vi "Memory Manager Pre-Build.vi"   [LabVIEW 2016]
uses:
  Build Automation.lvlib
types:
  T1 = cluster{"Status Message":refnum<data-value>, "Progress":refnum<data-value>, "Stop":refnum<data-value>}
  T2 = enum16{"Share clones between instances", "Preallocate clone for each instance"}
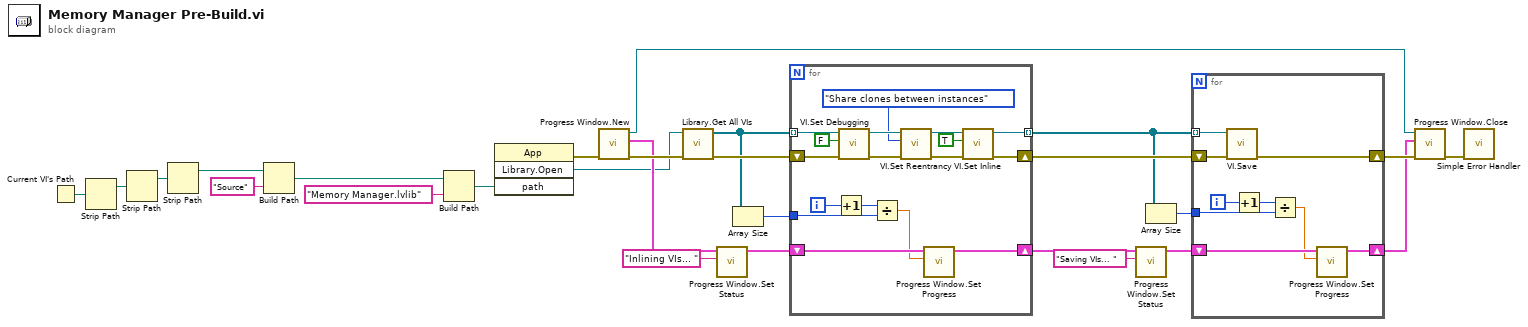
[diagram p0: block diagram]
diagram:
  n1 = Current VI's Path() -> (path=w26:path)
  n2 = Strip Path(path=w26) -> (stripped path=w25:path)  [unwired: 1 out]
  n3 = Strip Path(path=w25) -> (stripped path=w24:path)  [unwired: 1 out]
  n4 = Strip Path(path=w24) -> (stripped path=w23:path)  [unwired: 1 out]
  n5 = Build Path(base path=w23, name or relative path="Source") -> (appended path=w22:path)
  n6 = Build Path(base path=w22, name or relative path="Memory Manager.lvlib" ("library name")) -> (appended path=w20:path)
  n7 = invoke class="App" method="Library.Open"("path"=w20) -> (error out=w18:errorcluster, "Open Library"=w6:refnum<vi>)  [unwired: 3 in, 2 out]
  n8 = call "Progress Window.New.vi"("error in (no error)"=w18) -> ("error out"=w8:errorcluster, "DVRs"=w7:T1, "VI refnum"=w12:refnum<vi>)  [unwired: 8 in]
  n9 = call "Library.Get All VIs.vi"("error in (no error)"=w8, "library ref"=w6) -> ("error out"=w19:errorcluster, "vi refs"=w16:refnum<vi>[])  [unwired: 8 in]
  n10 = call "Progress Window.Set Status.vi"("Status Message"="Inlining VIs... " ("data value"), "DVRs in"=w7) -> ("DVRs out"=w14:T1)  [unwired: 8 in, 1 out]
  n11 = Array Size(array=w16) -> (size(s)=w15:i32)
  n12 = for {
    tunnel: w16 -> [w44] mode=indexing
    shift-right: [w28] -> w11
    shift-left: w19 -> [w43]
    tunnel: w15 -> [w34]
    shift-right: [w31] -> w10
    shift-left: w14 -> [w33]
    tunnel: [w29] -> w4 mode=indexing
    i -> [w36]
    n13 = Increment(x=w36) -> (x+1=w35:i32)
    n14 = call "VI.Set Debugging.vi"("error in (no error)"=w43, "Allow Debugging"=FALSE, "vi ref in"=w44) -> ("error out"=w40:errorcluster, "vi ref out"=w41:refnum<vi>)  [unwired: 7 in]
    n15 = Divide(x=w35, y=w34) -> (x/y=w32:dbl)
    n16 = call "VI.Set Reentrancy.vi"("error in (no error)"=w40, "Reentrancy Type"=T2."Share clones between instances", "vi ref in"=w41) -> ("error out"=w38:errorcluster, "vi ref out"=w39:refnum<vi>)  [unwired: 7 in]
    n17 = call "Progress Window.Set Progress.vi"("Progress"=w32, "DVRs in"=w33) -> ("DVRs out"=w31:T1)  [unwired: 8 in, 1 out]
    n18 = call "VI.Set Inline.vi"("error in (no error)"=w38, "Inline VI"=TRUE, "vi ref in"=w39) -> ("error out"=w28:errorcluster, "vi ref out"=w29:refnum<vi>)  [unwired: 7 in]
  }
  n19 = call "Progress Window.Set Status.vi"("Status Message"="Saving VIs... ", "DVRs in"=w10) -> ("DVRs out"=w5:T1)  [unwired: 8 in, 1 out]
  n20 = Array Size(array=w4) -> (size(s)=w3:i32)
  n21 = for {
    shift-right: [w51] -> w2
    shift-left: w11 -> [w53]
    tunnel: w4 -> [w52] mode=indexing
    shift-right: [w45] -> w1
    shift-left: w5 -> [w47]
    tunnel: w3 -> [w49]
    i -> [w48]
    n22 = call "VI.Save.vi"("error in (no error)"=w53, "vi ref in"=w52) -> ("error out"=w51:errorcluster)  [unwired: 8 in, 1 out]
    n23 = Increment(x=w48) -> (x+1=w50:i32)
    n24 = Divide(x=w50, y=w49) -> (x/y=w46:dbl)
    n25 = call "Progress Window.Set Progress.vi"("Progress"=w46, "DVRs in"=w47) -> ("DVRs out"=w45:T1)  [unwired: 8 in, 1 out]
  }
  n26 = call "Progress Window.Close.vi"("error in (no error)"=w2, "DVRs in"=w1, "VI refnum"=w12) -> ("error out"=w13:errorcluster)  [unwired: 8 in]
  n27 = call <vilib>:"Simple Error Handler.vi"("error in (no error)"=w13) -> ()  [unwired: 4 in, 5 out]
